vi "Clear Data.vi"() -> (3 "Success":bool)   [LabVIEW 2023]
doc: "HTTP Method VI that clears the weather data."
uses:
  Application/Weather Data.lvlib
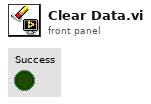
[diagram p1: front panel]
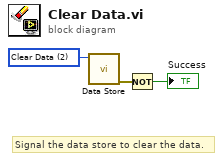
[diagram p0: block diagram]
diagram:
  w2 = u16 2 items=["Initialize Data Store", "Destroy Data Store", "Clear Data", "Append Data", "Get Last Data", "Get All Data"] ("action")
  # "Signal the data store to clear the data."
  n1 = call "Data Store.vi"("action"=w2) -> ("error out"=w1:errorcluster)  [unwired: 9 in, 1 out]
  n2 = Not(x=w1) -> (.not. x?=→"Success":bool)
